vi "cg_fid_V1.2.1.vi"() -> ()   [LabVIEW 2011]
panel:
  in  "stop":bool
  out "Start Indicator":bool
  in  "start chromat":bool
  in  "Abort Chrom":bool
  out "FID":cluster{"value":dbl}(graph)
  out "Temp History":cluster{"value":dbl}(graph)
  out "Time (min)":dbl
  out "Counter":i32
  in  "Stop Time (min)":dbl=15.0
  out "Time has Elapsed":bool
  in  "Start Button":bool
  out "TCD":dbl(graph)
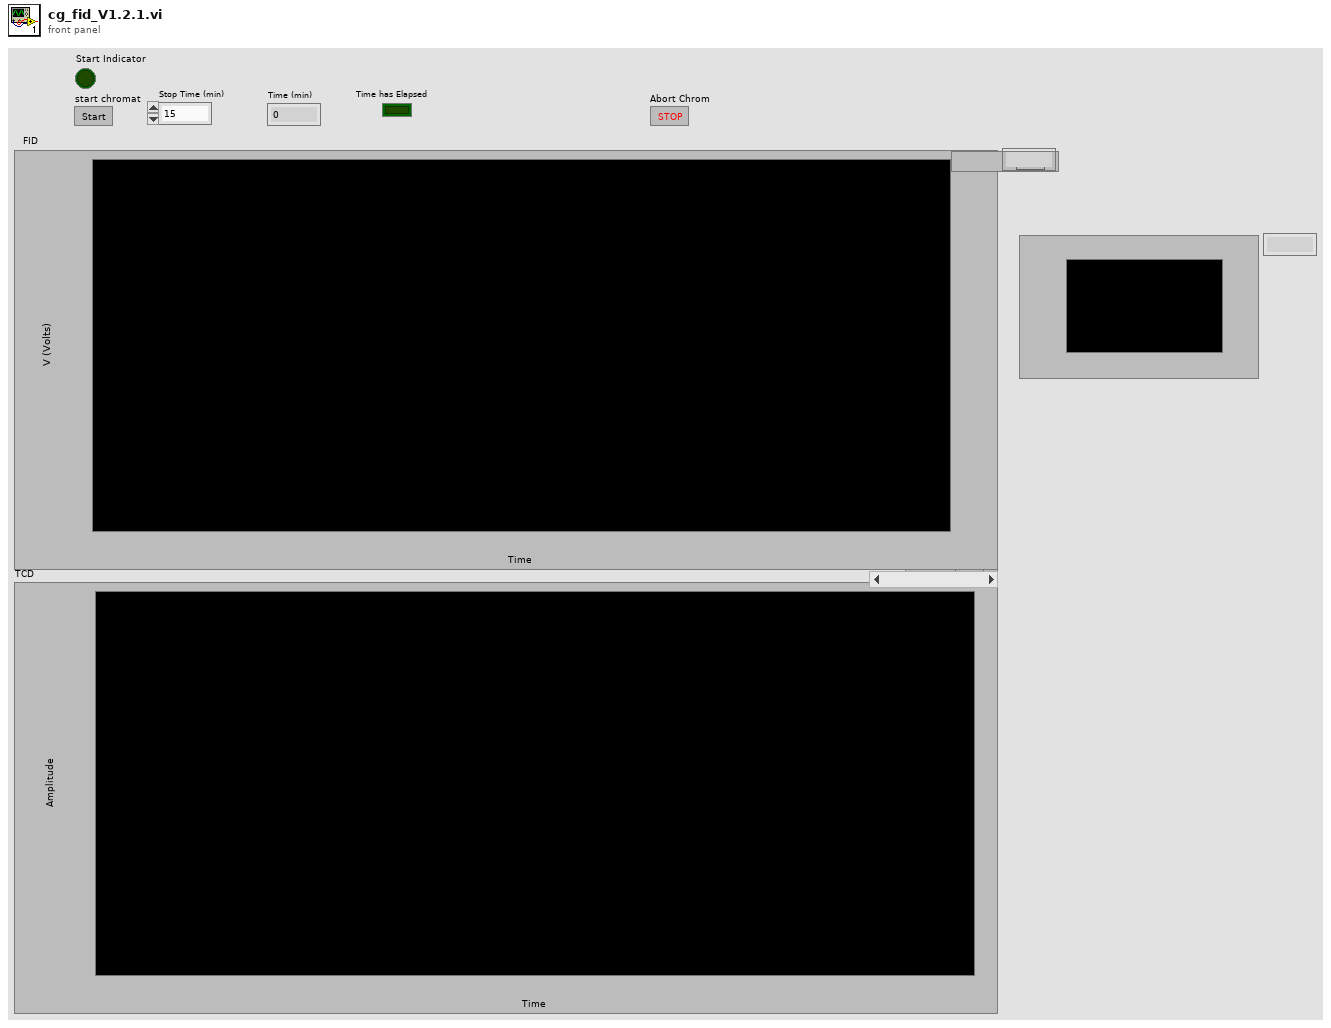
[diagram p1: front panel]
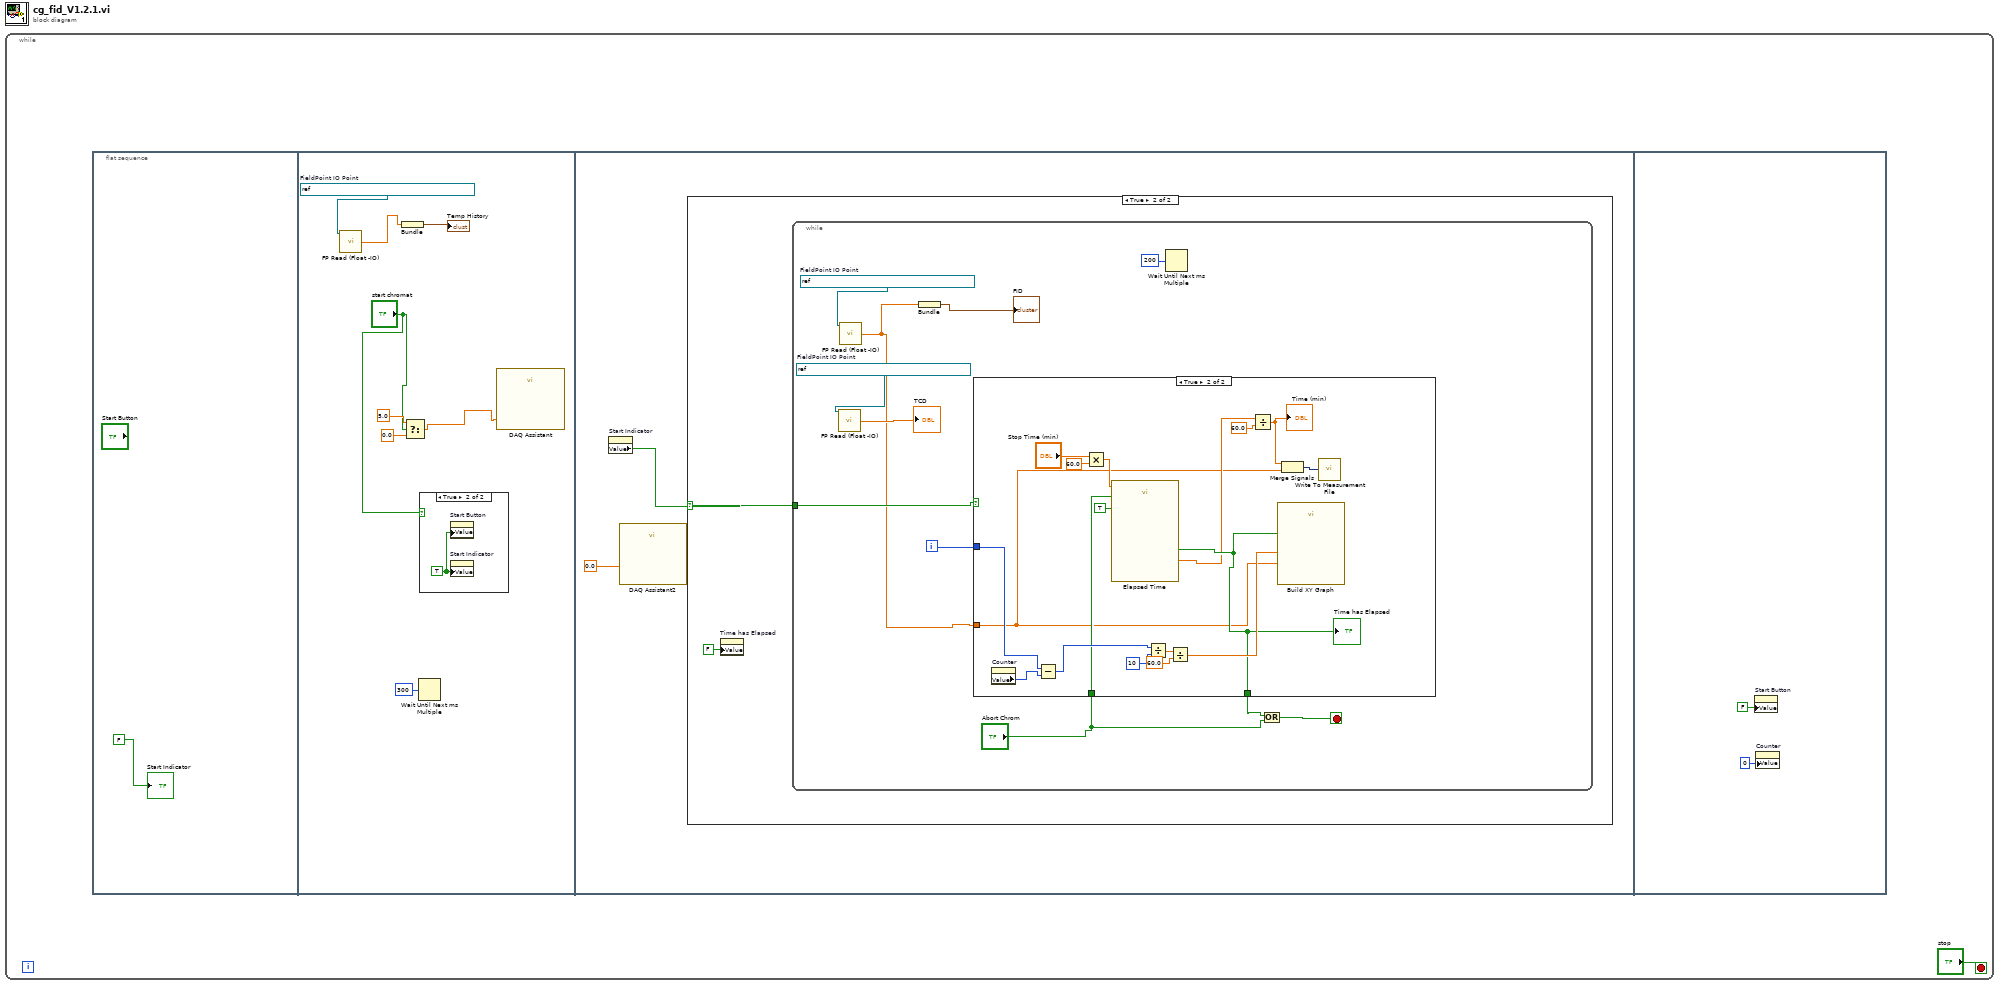
[diagram p0: block diagram]
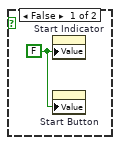
[diagram p2: hidden frame]
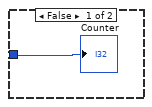
[diagram p4: hidden frame]
diagram:
  n1 = while {
    stop <- "stop" stop-if-true
    n2 = flat-sequence {
      frame #0 {
        "Start Indicator" <- FALSE
      }
      frame #1 {
        w5 = refnum<k21> "FieldPoint\\cfp2220\\cFP-AI-110 @4\\Channel 0"  # FieldPoint IO Point
        n3 = call <vilib>:"FP Read (Float -IO).vi"("FieldPoint IO Point In"=w5) -> ("value"=w4:dbl)  [unwired: 11 in, 3 out]
        n4 = Bundle("value"=w4) -> (→"Temp History":cluster{"value":dbl})  [unwired: 1 out]
        n5 = Select(t=5.0, s="start chromat", f=0.0) -> (s? t:f=w6:dbl)
        n6 = Wait Until Next ms Multiple(millisecond multiple=u32 300) -> ()  [unwired: 1 out]
        n7 = case shown="True" "start chromat" {
          frame False {
            w11 = FALSE ("Start Button")
            n8 = property on="Start Indicator" class="Bool (strict)"("Value"=w11) -> ()  [unwired: 2 in, 2 out]
            n9 = property on="Start Button" class="Bool (strict)"("Value"=w11) -> ()  [unwired: 2 in, 2 out]
          }
          frame True {
            w12 = TRUE ("Start Button")
            n10 = property on="Start Button" class="Bool (strict)"("Value"=w12) -> ()  [unwired: 2 in, 2 out]
            n11 = property on="Start Indicator" class="Bool (strict)"("Value"=w12) -> ()  [unwired: 2 in, 2 out]
          }
        }
        n12 = call "DAQ Assistant"("data"=w6) -> ()  [unwired: 17 in, 2 out]
      }
      frame #2 {
        n13 = property on="Start Indicator" class="Bool (strict)"() -> ("Value"=w14:bool)  [unwired: 2 in, 2 out]
        n14 = call "DAQ Assistant2"("data"=0.0 ("f")) -> ()  [unwired: 17 in, 2 out]
        n15 = case shown="True" w14 {
          selector: w14 -> [_ w16]
          frame False {
          }
          frame True {
            n16 = property on="Time has Elapsed" class="Bool (strict)"("Value"=FALSE ("Time has Elapsed")) -> ()  [unwired: 2 in, 2 out]
            n17 = while {
              tunnel: w16 -> [w21]
              i -> [w23]
              stop <- w18 stop-if-true
              w26 = refnum<k21> "FieldPoint\\cfp2220\\cFP-AI-110 @4\\Channel 2"  # FieldPoint IO Point
              w27 = refnum<k21> "FieldPoint\\cfp2220\\cFP-AI-110 @4\\Channel 0"  # FieldPoint IO Point
              n18 = call <vilib>:"FP Read (Float -IO).vi"("FieldPoint IO Point In"=w26) -> ("value"=→"TCD":dbl)  [unwired: 11 in, 3 out]
              n19 = call <vilib>:"FP Read (Float -IO).vi"("FieldPoint IO Point In"=w27) -> ("value"=w19:dbl)  [unwired: 11 in, 3 out]
              n20 = Bundle("value"=w19) -> (→"FID":cluster{"value":dbl})  [unwired: 1 out]
              n21 = case shown="True" w21 {
                tunnel: w19 -> [_ w29]
                tunnel: w23 -> [w28 w42]
                tunnel: [_ w34] -> w20
                tunnel: "Abort Chrom" -> [_ w30]
                frame False {
                  "Counter" <- w28
                }
                frame True {
                  n22 = property on="Counter" class="DigNum (strict)"() -> ("Value"=w41:i32)  [unwired: 2 in, 2 out]
                  n23 = Subtract(x=w42, y=w41) -> (x-y=w43:i32)
                  n24 = Multiply(x="Stop Time (min)", y=60.0) -> (x*y=w37:dbl)
                  n25 = call "Elapsed Time"("Time Target (s)"=w37, "Reset"=w30, "Auto Reset"=TRUE) -> ("Elapsed Time (s)"=w33:dbl, "Time has Elapsed"=w34:bool)  [unwired: 9 in, 6 out]
                  "Time has Elapsed" <- w34
                  n26 = Divide(x=w43, y=10) -> (x/y=w45:dbl)
                  n27 = Divide(x=w45, y=60.0) -> (x/y=w40:dbl)
                  n28 = Divide(x=w33, y=60.0) -> (x/y=w32:dbl)
                  "Time (min)" <- w32
                  n29 = call "Build XY Graph"("Enable"=w34, "Y Input"=w29, "X Input"=w40) -> ()  [unwired: 2 in, 7 out]
                  n30 = Merge Signals(w32, w29) -> (w38:dynamicdata)
                  n31 = call "Write To Measurement File"("Signals"=w38) -> ()  [unwired: 16 in, 3 out]
                }
              }
              n32 = Wait Until Next ms Multiple(millisecond multiple=u32 200) -> ()  [unwired: 1 out]
              n33 = Or(x=w20, y="Abort Chrom") -> (x .or. y?=w18:bool)
            }
          }
        }
      }
      frame #3 {
        n34 = property on="Start Button" class="Bool (strict)"("Value"=FALSE ("Start Button")) -> ()  [unwired: 2 in, 2 out]
        n35 = property on="Counter" class="DigNum (strict)"("Value"=0 ("Numeric")) -> ()  [unwired: 2 in, 2 out]
      }
    }
  }
